vi "Spindle_load_RT_1 (SubVI).vi"(9 "?":T1, 10 "concatenated string 4":string, 11 "String":string) -> (0 "error out":errorcluster, 1 "content 4":string, 2 "content1 2":string, 3 "output cluster":T1, 4 "empty? 2":bool, 5 "concatenated string":string, 6 "load":string, 7 "concatenated string 2":string)   [LabVIEW 2017]
uses:
  MT_connect_data.ctl
  <vilib>/regexp/Match Regular Expression.xnode
  <vilib>/addons/internet/NI_InternetTK_Core_VIs.lvlib
panel:
  out "Position A 2":string
  out "content 7":string
  out "content 6":string
  out "after match":string
  out "Z_position":string
  out "Z_load":string
  out "Y_load":string
  out "X_position":string
  out "X_load":string
  out "Y_poistion":string
  out "K_position":string
  out "J_position":string
  out "I_position":string
  out "concatenated string 6":string
  out "content 3":string
  out "Position B":string
  out "B_load":string
  out "A_Load":string
  out "content 2":string
  out "concatenated string 5":string
  out "Position A":string
  out "Avail":string
  out "Tool_ID":string
  out "Program_name":string
  out "Controller_Mode":string
  out "Line_code":string
  out "program_status":string
  out "Block":string
  out "feeover":string
  out "Speedover":string
  out "path feedrate":string
  out "content":string
  out "error out 2":errorcluster
  out "spindle speed":string
  out "content 5":string
  out "empty? 3":bool
  out "after match 3":string
  out "content1 3":string
  out "concatenated string 3":string
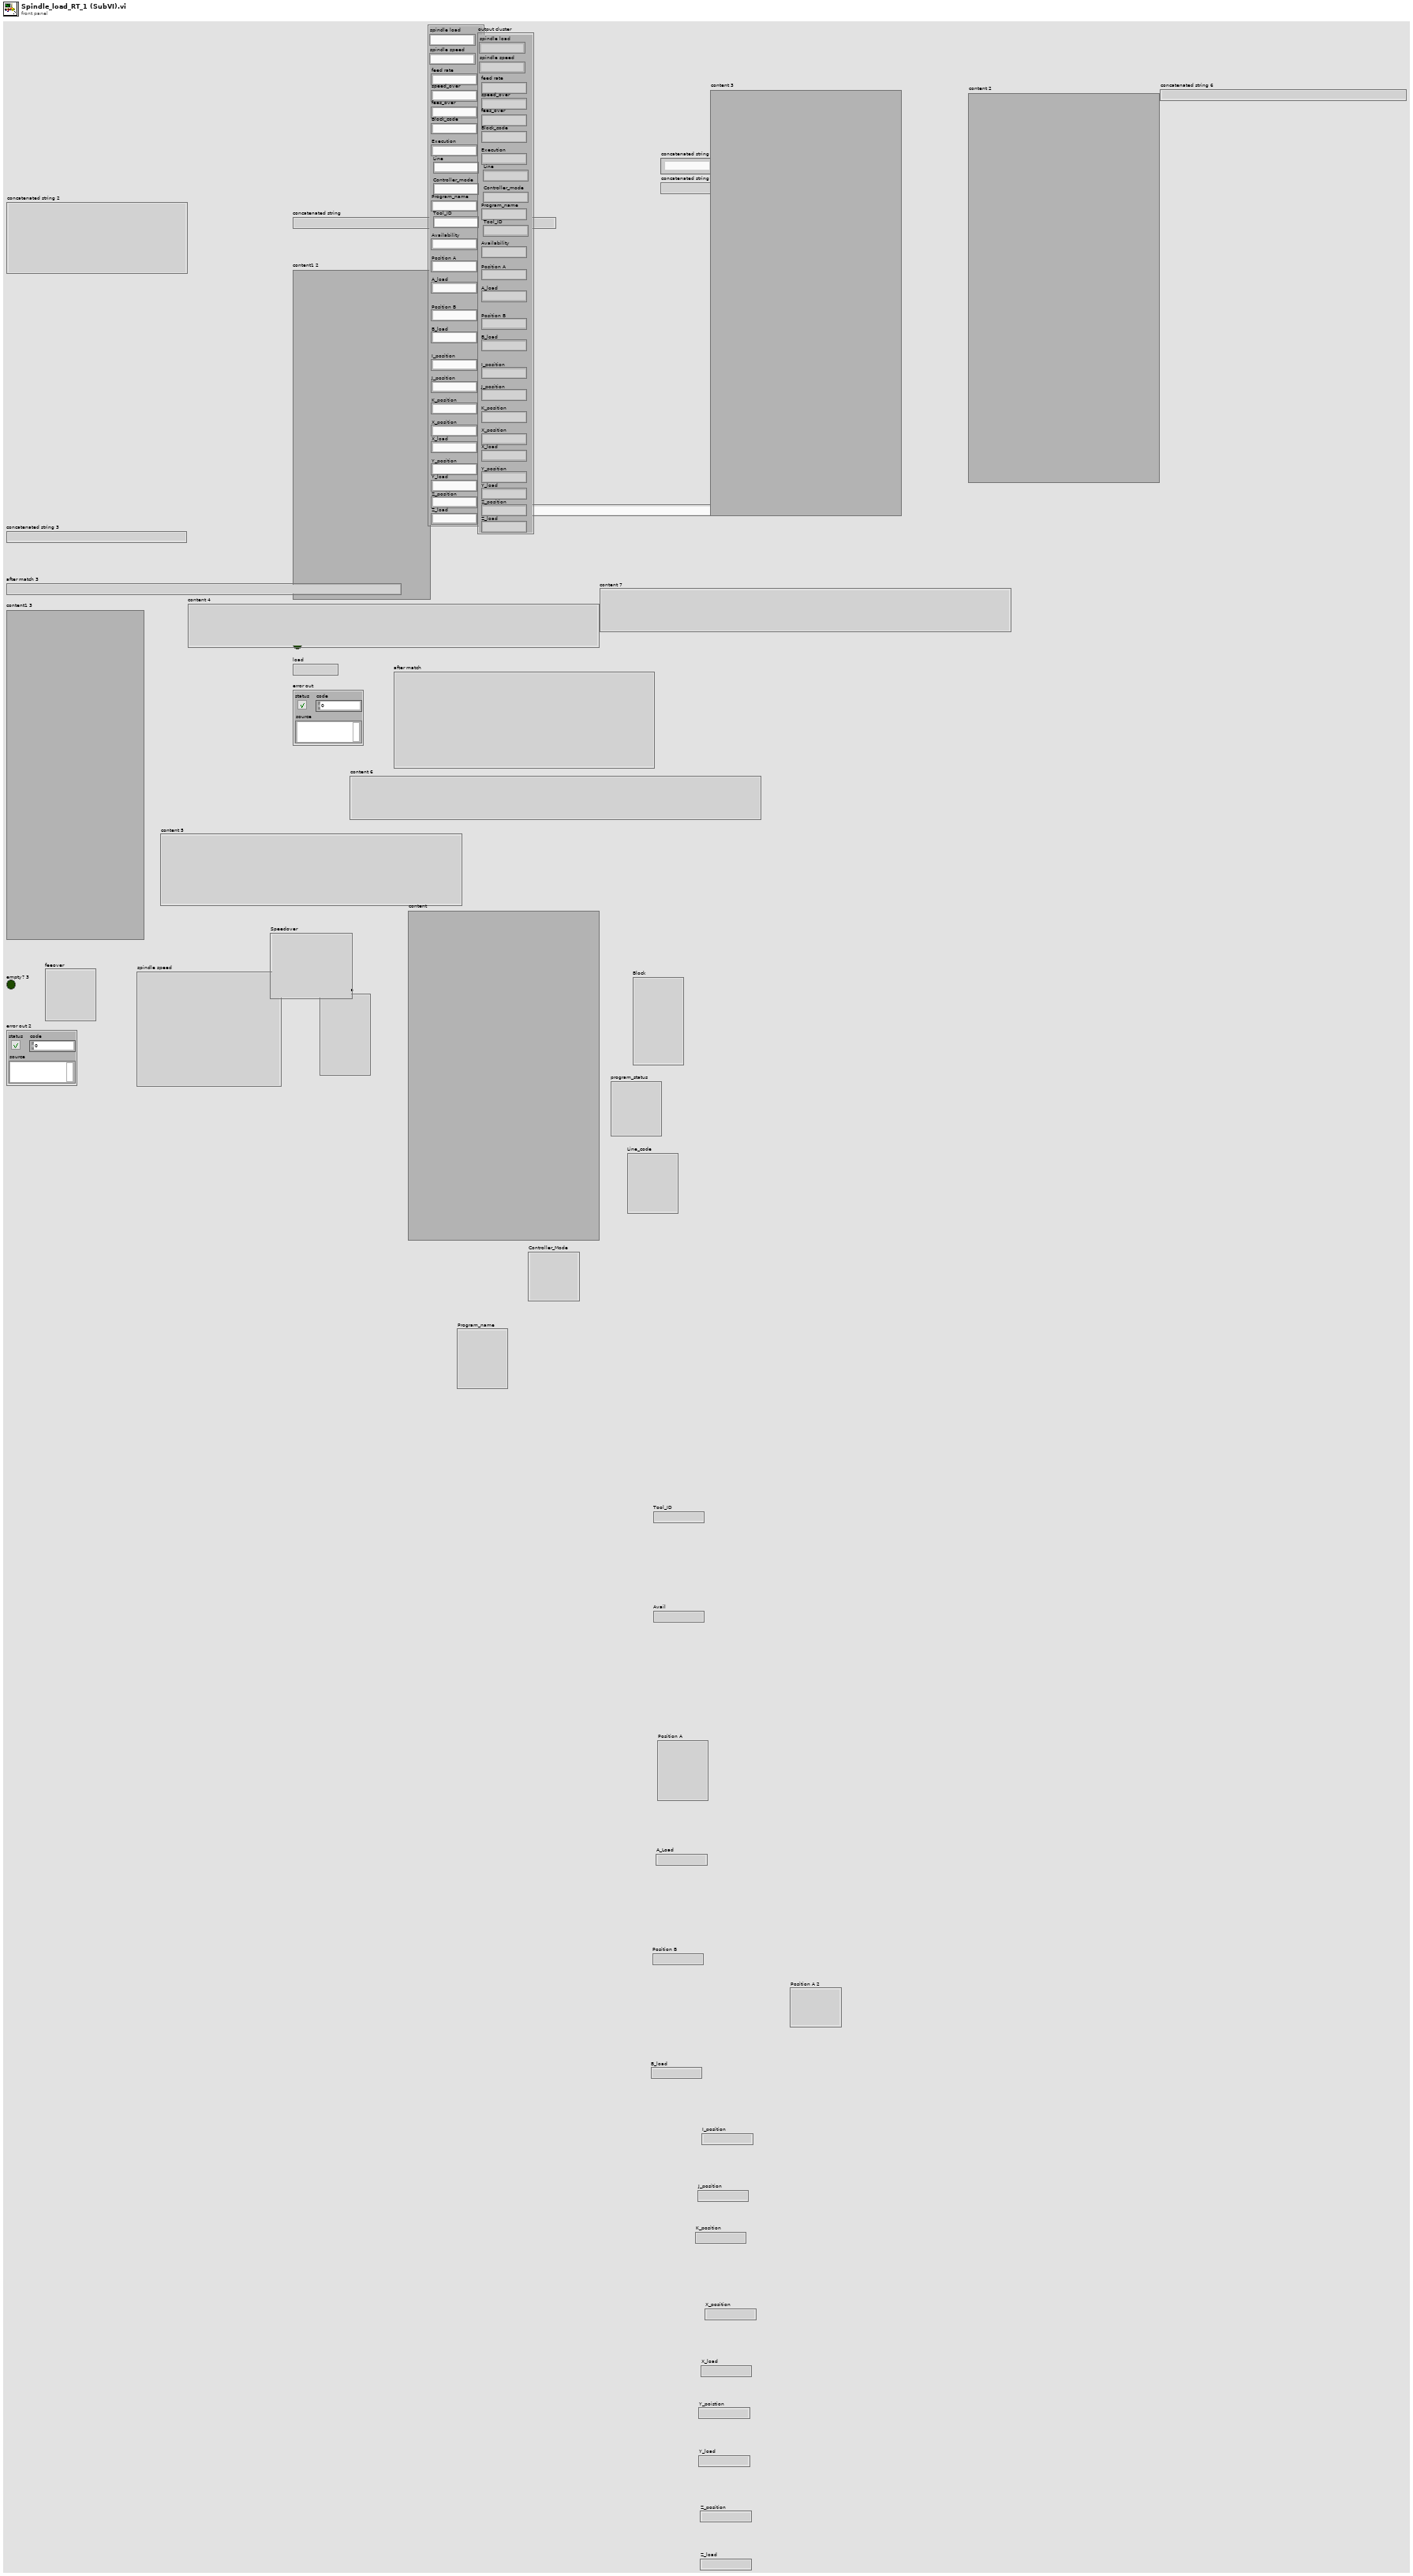
[diagram p1: front panel]
types:
  T1 = typedef "MT_connect_data.ctl" = cluster{"spindle load ":string, "spindle speed ":string, "feed rate":string, "speed_over":string, "fees_over":string, "Block_code":string, "Execution":string, "Line":string, "Controller_mode":string, "Program_name":string, "Tool_ID":string, "Availability":string, "Position A":string, "A_load":string, "Position B":string, "B_load":string, "I_position":string, "J_position":string, "K_position":string, "X_position":string, "X_load":string, "Y_position":string, "Y_load":string, "Z_position":string, "Z_load":string}
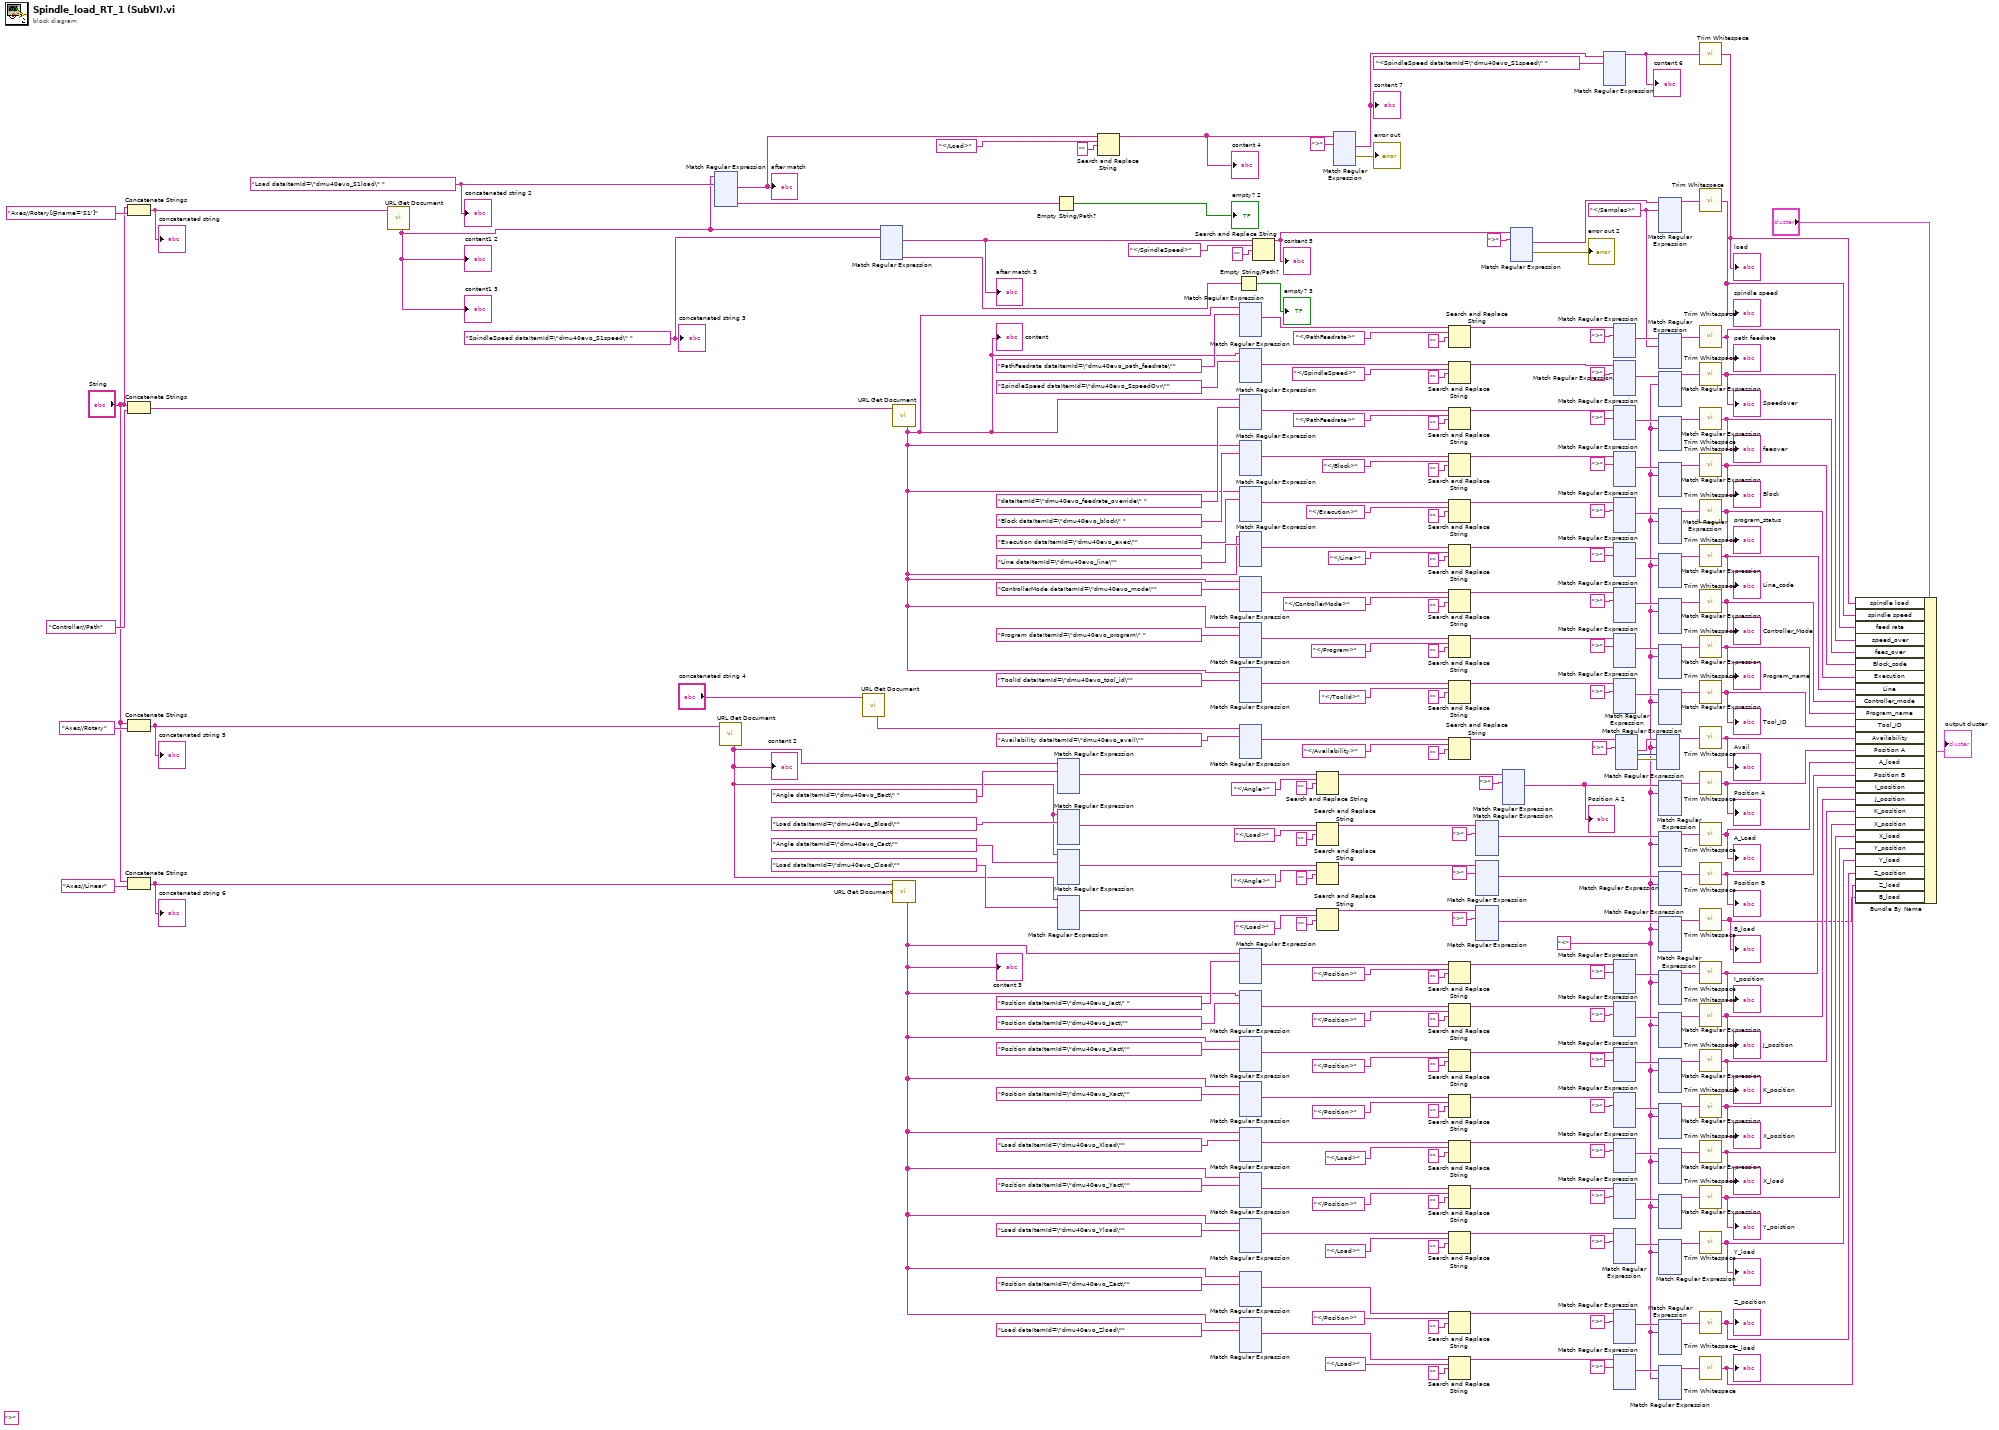
[diagram p0: block diagram]
diagram:
  w4 = "<" ("string")
  w55 = "</Samples>" ("string")
  (unwired) ">" ("string")
  w241 = "SpindleSpeed dataItemId=\"dmu40evo_S1speed\" " ("regular expression")
  w252 = "Load dataItemId=\"dmu40evo_S1load\" " ("regular expression")
  n1 = Concatenate Strings("String", "Axes//Rotary[@name='S1']" ("string")) -> (w247:string)
  "concatenated string" <- w247
  n2 = Concatenate Strings("String", "Controller//Path" ("string")) -> (w228:string)
  n3 = Concatenate Strings("String", "Axes//Rotary" ("string")) -> (w127:string)
  "concatenated string 5" <- w127
  n4 = Concatenate Strings("String", "Axes//Linear" ("string")) -> (w126:string)
  "concatenated string 6" <- w126
  n5 = call <vilib>:"URL Get Document.vi"("URL"=w247) -> ("content"=w233:string)  [unwired: 6 in, 4 out]
  "content1 2" <- w233
  "content1 3" <- w233
  n6 = xnode "Match Regular Expression"("input string"=w233, "regular expression"=w252) -> ("after match"=w244:string, "submatch 1"=w246:string)  [unwired: 4 in, 4 out]
  "after match" <- w244
  n7 = call <vilib>:"URL Get Document.vi"("URL"=w127) -> ("content"=w131:string)  [unwired: 6 in, 4 out]
  "content 2" <- w131
  n8 = call <vilib>:"URL Get Document.vi"("URL"="concatenated string 4") -> ("content"=w163:string)  [unwired: 6 in, 4 out]
  n9 = xnode "Match Regular Expression"("input string"=w233, "regular expression"=w241) -> ("after match"=w235:string, "submatch 1"=w237:string)  [unwired: 4 in, 4 out]
  "after match 3" <- w235
  n10 = call <vilib>:"URL Get Document.vi"("URL"=w228) -> ("content"=w162:string)  [unwired: 6 in, 4 out]
  "content" <- w162
  n11 = call <vilib>:"URL Get Document.vi"("URL"=w126) -> ("content"=w70:string)  [unwired: 6 in, 4 out]
  "content 3" <- w70
  n12 = Empty String/Path?(string/path=w246) -> (empty?=→"empty? 2":bool)
  n13 = xnode "Match Regular Expression"("input string"=w131, "regular expression"="Angle dataItemId=\"dmu40evo_Bact\" ") -> ("after match"=w155:string)  [unwired: 4 in, 5 out]
  n14 = xnode "Match Regular Expression"("input string"=w131, "regular expression"="Load dataItemId=\"dmu40evo_Bload\"") -> ("after match"=w145:string)  [unwired: 4 in, 5 out]
  n15 = xnode "Match Regular Expression"("input string"=w131, "regular expression"="Angle dataItemId=\"dmu40evo_Cact\"") -> ("after match"=w133:string)  [unwired: 4 in, 5 out]
  n16 = xnode "Match Regular Expression"("input string"=w131, "regular expression"="Load dataItemId=\"dmu40evo_Cload\"") -> ("after match"=w142:string)  [unwired: 4 in, 5 out]
  n17 = Search and Replace String(input string=w244, search string="</Load>" ("string"), replace string="" ("string")) -> (result string=w243:string)  [unwired: 5 in, 3 out]
  "content 4" <- w243
  n18 = Empty String/Path?(string/path=w237) -> (empty?=→"empty? 3":bool)
  n19 = xnode "Match Regular Expression"("input string"=w162, "regular expression"="PathFeedrate dataItemId=\"dmu40evo_path_feedrate\"") -> ("after match"=w226:string)  [unwired: 4 in, 5 out]
  n20 = xnode "Match Regular Expression"("input string"=w162, "regular expression"="SpindleSpeed dataItemId=\"dmu40evo_SspeedOvr\"") -> ("after match"=w214:string)  [unwired: 4 in, 5 out]
  n21 = xnode "Match Regular Expression"("input string"=w162, "regular expression"="dataItemId=\"dmu40evo_feedrate_override\" ") -> ("after match"=w213:string)  [unwired: 4 in, 5 out]
  n22 = xnode "Match Regular Expression"("input string"=w162, "regular expression"="Block dataItemId=\"dmu40evo_block\" ") -> ("after match"=w200:string)  [unwired: 4 in, 5 out]
  n23 = xnode "Match Regular Expression"("input string"=w162, "regular expression"="Execution dataItemId=\"dmu40evo_exec\"") -> ("after match"=w192:string)  [unwired: 4 in, 5 out]
  n24 = xnode "Match Regular Expression"("input string"=w162, "regular expression"="Line dataItemId=\"dmu40evo_line\"") -> ("after match"=w191:string)  [unwired: 4 in, 5 out]
  n25 = xnode "Match Regular Expression"("input string"=w162, "regular expression"="ControllerMode dataItemId=\"dmu40evo_mode\"") -> ("after match"=w187:string)  [unwired: 4 in, 5 out]
  n26 = xnode "Match Regular Expression"("input string"=w162, "regular expression"="Program dataItemId=\"dmu40evo_program\" ") -> ("after match"=w178:string)  [unwired: 4 in, 5 out]
  n27 = xnode "Match Regular Expression"("input string"=w162, "regular expression"="ToolId dataItemId=\"dmu40evo_tool_id\"") -> ("after match"=w175:string)  [unwired: 4 in, 5 out]
  n28 = xnode "Match Regular Expression"("input string"=w163, "regular expression"="Availability dataItemId=\"dmu40evo_avail\"") -> ("after match"=w166:string)  [unwired: 4 in, 5 out]
  n29 = xnode "Match Regular Expression"("input string"=w70, "regular expression"="Position dataItemId=\"dmu40evo_Iact\" ") -> ("after match"=w120:string)  [unwired: 4 in, 5 out]
  n30 = xnode "Match Regular Expression"("input string"=w70, "regular expression"="Position dataItemId=\"dmu40evo_Jact\"") -> ("after match"=w117:string)  [unwired: 4 in, 5 out]
  n31 = xnode "Match Regular Expression"("input string"=w70, "regular expression"="Position dataItemId=\"dmu40evo_Kact\"") -> ("after match"=w108:string)  [unwired: 4 in, 5 out]
  n32 = xnode "Match Regular Expression"("input string"=w70, "regular expression"="Position dataItemId=\"dmu40evo_Xact\"") -> ("after match"=w93:string)  [unwired: 4 in, 5 out]
  n33 = xnode "Match Regular Expression"("input string"=w70, "regular expression"="Load dataItemId=\"dmu40evo_Xload\"") -> ("after match"=w96:string)  [unwired: 4 in, 5 out]
  n34 = xnode "Match Regular Expression"("input string"=w70, "regular expression"="Position dataItemId=\"dmu40evo_Yact\"") -> ("after match"=w105:string)  [unwired: 4 in, 5 out]
  n35 = xnode "Match Regular Expression"("input string"=w70, "regular expression"="Load dataItemId=\"dmu40evo_Yload\"") -> ("after match"=w84:string)  [unwired: 4 in, 5 out]
  n36 = xnode "Match Regular Expression"("input string"=w70, "regular expression"="Position dataItemId=\"dmu40evo_Zact\"") -> ("after match"=w72:string)  [unwired: 4 in, 5 out]
  n37 = xnode "Match Regular Expression"("input string"=w70, "regular expression"="Load dataItemId=\"dmu40evo_Zload\"") -> ("after match"=w81:string)  [unwired: 4 in, 5 out]
  n38 = Search and Replace String(input string=w235, search string="</SpindleSpeed>" ("string"), replace string="" ("string")) -> (result string=w234:string)  [unwired: 5 in, 3 out]
  "content 5" <- w234
  n39 = Search and Replace String(input string=w155, search string="</Angle>" ("string"), replace string="" ("string")) -> (result string=w156:string)  [unwired: 5 in, 3 out]
  n40 = Search and Replace String(input string=w145, search string="</Load>" ("string"), replace string="" ("string")) -> (result string=w144:string)  [unwired: 5 in, 3 out]
  n41 = Search and Replace String(input string=w133, search string="</Angle>" ("string"), replace string="" ("string")) -> (result string=w132:string)  [unwired: 5 in, 3 out]
  n42 = Search and Replace String(input string=w142, search string="</Load>" ("string"), replace string="" ("string")) -> (result string=w143:string)  [unwired: 5 in, 3 out]
  n43 = xnode "Match Regular Expression"("input string"=w243, "regular expression"=">" ("string")) -> ("after match"=w59:string, "error out"=→"error out":errorcluster)  [unwired: 4 in, 4 out]
  "content 7" <- w59
  n44 = Search and Replace String(input string=w226, search string="</PathFeedrate>" ("string"), replace string="" ("string")) -> (result string=w221:string)  [unwired: 5 in, 3 out]
  n45 = Search and Replace String(input string=w214, search string="</SpindleSpeed>" ("string"), replace string="" ("string")) -> (result string=w219:string)  [unwired: 5 in, 3 out]
  n46 = Search and Replace String(input string=w213, search string="</PathFeedrate>" ("string"), replace string="" ("string")) -> (result string=w208:string)  [unwired: 5 in, 3 out]
  n47 = Search and Replace String(input string=w200, search string="</Block>" ("string"), replace string="" ("string")) -> (result string=w205:string)  [unwired: 5 in, 3 out]
  n48 = Search and Replace String(input string=w192, search string="</Execution>" ("string"), replace string="" ("string")) -> (result string=w190:string)  [unwired: 5 in, 3 out]
  n49 = Search and Replace String(input string=w191, search string="</Line>" ("string"), replace string="" ("string")) -> (result string=w189:string)  [unwired: 5 in, 3 out]
  n50 = Search and Replace String(input string=w187, search string="</ControllerMode>" ("string"), replace string="" ("string")) -> (result string=w188:string)  [unwired: 5 in, 3 out]
  n51 = Search and Replace String(input string=w178, search string="</Program>" ("string"), replace string="" ("string")) -> (result string=w177:string)  [unwired: 5 in, 3 out]
  n52 = Search and Replace String(input string=w175, search string="</ToolId>" ("string"), replace string="" ("string")) -> (result string=w176:string)  [unwired: 5 in, 3 out]
  n53 = Search and Replace String(input string=w166, search string="</Availability>" ("string"), replace string="" ("string")) -> (result string=w165:string)  [unwired: 5 in, 3 out]
  n54 = Search and Replace String(input string=w120, search string="</Position>" ("string"), replace string="" ("string")) -> (result string=w119:string)  [unwired: 5 in, 3 out]
  n55 = Search and Replace String(input string=w117, search string="</Position>" ("string"), replace string="" ("string")) -> (result string=w118:string)  [unwired: 5 in, 3 out]
  n56 = Search and Replace String(input string=w108, search string="</Position>" ("string"), replace string="" ("string")) -> (result string=w107:string)  [unwired: 5 in, 3 out]
  n57 = Search and Replace String(input string=w93, search string="</Position>" ("string"), replace string="" ("string")) -> (result string=w94:string)  [unwired: 5 in, 3 out]
  n58 = Search and Replace String(input string=w96, search string="</Load>" ("string"), replace string="" ("string")) -> (result string=w95:string)  [unwired: 5 in, 3 out]
  n59 = Search and Replace String(input string=w105, search string="</Position>" ("string"), replace string="" ("string")) -> (result string=w106:string)  [unwired: 5 in, 3 out]
  n60 = Search and Replace String(input string=w84, search string="</Load>" ("string"), replace string="" ("string")) -> (result string=w83:string)  [unwired: 5 in, 3 out]
  n61 = Search and Replace String(input string=w72, search string="</Position>" ("string"), replace string="" ("string")) -> (result string=w71:string)  [unwired: 5 in, 3 out]
  n62 = Search and Replace String(input string=w81, search string="</Load>" ("string"), replace string="" ("string")) -> (result string=w82:string)  [unwired: 5 in, 3 out]
  n63 = xnode "Match Regular Expression"("input string"=w144, "regular expression"=">" ("string")) -> ("after match"=w35:string)  [unwired: 4 in, 5 out]
  n64 = xnode "Match Regular Expression"("input string"=w132, "regular expression"=">" ("string")) -> ("after match"=w34:string)  [unwired: 4 in, 5 out]
  n65 = xnode "Match Regular Expression"("input string"=w143, "regular expression"=">" ("string")) -> ("after match"=w33:string)  [unwired: 4 in, 5 out]
  n66 = xnode "Match Regular Expression"("input string"=w156, "regular expression"=">" ("string")) -> ("after match"=w23:string)  [unwired: 4 in, 5 out]
  "Position A 2" <- w23
  n67 = xnode "Match Regular Expression"("input string"=w234, "regular expression"=">" ("string")) -> ("after match"=w58:string, "error out"=→"error out 2":errorcluster)  [unwired: 4 in, 4 out]
  n68 = xnode "Match Regular Expression"("input string"=w59, "regular expression"="<SpindleSpeed dataItemId=\"dmu40evo_S1speed\" ") -> ("before match"=w60:string)  [unwired: 4 in, 5 out]
  "content 6" <- w60
  n69 = xnode "Match Regular Expression"("input string"=w221, "regular expression"=">" ("string")) -> ("after match"=w56:string)  [unwired: 4 in, 5 out]
  n70 = xnode "Match Regular Expression"("input string"=w219, "regular expression"=">" ("string")) -> ("after match"=w49:string)  [unwired: 4 in, 5 out]
  n71 = xnode "Match Regular Expression"("input string"=w208, "regular expression"=">" ("string")) -> ("after match"=w5:string)  [unwired: 4 in, 5 out]
  n72 = xnode "Match Regular Expression"("input string"=w205, "regular expression"=">" ("string")) -> ("after match"=w8:string)  [unwired: 4 in, 5 out]
  n73 = xnode "Match Regular Expression"("input string"=w190, "regular expression"=">" ("string")) -> ("after match"=w51:string)  [unwired: 4 in, 5 out]
  n74 = xnode "Match Regular Expression"("input string"=w189, "regular expression"=">" ("string")) -> ("after match"=w47:string)  [unwired: 4 in, 5 out]
  n75 = xnode "Match Regular Expression"("input string"=w188, "regular expression"=">" ("string")) -> ("after match"=w45:string)  [unwired: 4 in, 5 out]
  n76 = xnode "Match Regular Expression"("input string"=w177, "regular expression"=">" ("string")) -> ("after match"=w39:string)  [unwired: 4 in, 5 out]
  n77 = xnode "Match Regular Expression"("input string"=w176, "regular expression"=">" ("string")) -> ("after match"=w38:string)  [unwired: 4 in, 5 out]
  n78 = xnode "Match Regular Expression"("input string"=w119, "regular expression"=">" ("string")) -> ("after match"=w32:string)  [unwired: 4 in, 5 out]
  n79 = xnode "Match Regular Expression"("input string"=w118, "regular expression"=">" ("string")) -> ("after match"=w31:string)  [unwired: 4 in, 5 out]
  n80 = xnode "Match Regular Expression"("input string"=w107, "regular expression"=">" ("string")) -> ("after match"=w30:string)  [unwired: 4 in, 5 out]
  n81 = xnode "Match Regular Expression"("input string"=w94, "regular expression"=">" ("string")) -> ("after match"=w29:string)  [unwired: 4 in, 5 out]
  n82 = xnode "Match Regular Expression"("input string"=w95, "regular expression"=">" ("string")) -> ("after match"=w28:string)  [unwired: 4 in, 5 out]
  n83 = xnode "Match Regular Expression"("input string"=w106, "regular expression"=">" ("string")) -> ("after match"=w27:string)  [unwired: 4 in, 5 out]
  n84 = xnode "Match Regular Expression"("input string"=w83, "regular expression"=">" ("string")) -> ("after match"=w26:string)  [unwired: 4 in, 5 out]
  n85 = xnode "Match Regular Expression"("input string"=w71, "regular expression"=">" ("string")) -> ("after match"=w25:string)  [unwired: 4 in, 5 out]
  n86 = xnode "Match Regular Expression"("input string"=w82, "regular expression"=">" ("string")) -> ("after match"=w24:string)  [unwired: 4 in, 5 out]
  n87 = xnode "Match Regular Expression"("input string"=w165, "regular expression"=">" ("string")) -> ("after match"=w37:string, "offset past match"=w41:i32, "error out"=w40:errorcluster)  [unwired: 4 in, 3 out]
  n88 = xnode "Match Regular Expression"("input string"=w37, "regular expression"=w4, "offset (0)"=w41, "error in"=w40) -> ("before match"=w22:string)  [unwired: 2 in, 5 out]
  n89 = xnode "Match Regular Expression"("input string"=w58, "regular expression"=w55) -> ("before match"=w57:string)  [unwired: 4 in, 5 out]
  n90 = xnode "Match Regular Expression"("input string"=w56, "regular expression"=w55) -> ("before match"=w54:string)  [unwired: 4 in, 5 out]
  n91 = xnode "Match Regular Expression"("input string"=w49, "regular expression"=w4) -> ("before match"=w53:string)  [unwired: 4 in, 5 out]
  n92 = xnode "Match Regular Expression"("input string"=w5, "regular expression"=w4) -> ("before match"=w6:string)  [unwired: 4 in, 5 out]
  n93 = xnode "Match Regular Expression"("input string"=w8, "regular expression"=w4) -> ("before match"=w7:string)  [unwired: 4 in, 5 out]
  n94 = xnode "Match Regular Expression"("input string"=w51, "regular expression"=w4) -> ("before match"=w50:string)  [unwired: 4 in, 5 out]
  n95 = xnode "Match Regular Expression"("input string"=w47, "regular expression"=w4) -> ("before match"=w46:string)  [unwired: 4 in, 5 out]
  n96 = xnode "Match Regular Expression"("input string"=w45, "regular expression"=w4) -> ("before match"=w44:string)  [unwired: 4 in, 5 out]
  n97 = xnode "Match Regular Expression"("input string"=w39, "regular expression"=w4) -> ("before match"=w43:string)  [unwired: 4 in, 5 out]
  n98 = xnode "Match Regular Expression"("input string"=w38, "regular expression"=w4) -> ("before match"=w42:string)  [unwired: 4 in, 5 out]
  n99 = xnode "Match Regular Expression"("input string"=w23, "regular expression"=w4) -> ("before match"=w21:string)  [unwired: 4 in, 5 out]
  n100 = xnode "Match Regular Expression"("input string"=w35, "regular expression"=w4) -> ("before match"=w20:string)  [unwired: 4 in, 5 out]
  n101 = xnode "Match Regular Expression"("input string"=w34, "regular expression"=w4) -> ("before match"=w19:string)  [unwired: 4 in, 5 out]
  n102 = xnode "Match Regular Expression"("input string"=w33, "regular expression"=w4) -> ("before match"=w18:string)  [unwired: 4 in, 5 out]
  n103 = xnode "Match Regular Expression"("input string"=w32, "regular expression"=w4) -> ("before match"=w17:string)  [unwired: 4 in, 5 out]
  n104 = xnode "Match Regular Expression"("input string"=w31, "regular expression"=w4) -> ("before match"=w16:string)  [unwired: 4 in, 5 out]
  n105 = xnode "Match Regular Expression"("input string"=w30, "regular expression"=w4) -> ("before match"=w15:string)  [unwired: 4 in, 5 out]
  n106 = xnode "Match Regular Expression"("input string"=w29, "regular expression"=w4) -> ("before match"=w14:string)  [unwired: 4 in, 5 out]
  n107 = xnode "Match Regular Expression"("input string"=w28, "regular expression"=w4) -> ("before match"=w13:string)  [unwired: 4 in, 5 out]
  n108 = xnode "Match Regular Expression"("input string"=w27, "regular expression"=w4) -> ("before match"=w12:string)  [unwired: 4 in, 5 out]
  n109 = xnode "Match Regular Expression"("input string"=w26, "regular expression"=w4) -> ("before match"=w11:string)  [unwired: 4 in, 5 out]
  n110 = xnode "Match Regular Expression"("input string"=w25, "regular expression"=w4) -> ("before match"=w10:string)  [unwired: 4 in, 5 out]
  n111 = xnode "Match Regular Expression"("input string"=w24, "regular expression"=w4) -> ("before match"=w9:string)  [unwired: 4 in, 5 out]
  n112 = call <vilib>:"Trim Whitespace.vi"("string"=w60) -> ("trimmed string"=w231:string)  [unwired: 1 in]
  "load" <- w231
  n113 = call <vilib>:"Trim Whitespace.vi"("string"=w57) -> ("trimmed string"=w230:string)  [unwired: 1 in]
  "spindle speed" <- w230
  n114 = call <vilib>:"Trim Whitespace.vi"("string"=w54) -> ("trimmed string"=w220:string)  [unwired: 1 in]
  "path feedrate" <- w220
  n115 = call <vilib>:"Trim Whitespace.vi"("string"=w53) -> ("trimmed string"=w207:string)  [unwired: 1 in]
  "Speedover" <- w207
  n116 = call <vilib>:"Trim Whitespace.vi"("string"=w6) -> ("trimmed string"=w206:string)  [unwired: 1 in]
  "feeover" <- w206
  n117 = call <vilib>:"Trim Whitespace.vi"("string"=w7) -> ("trimmed string"=w3:string)  [unwired: 1 in]
  "Block" <- w3
  n118 = call <vilib>:"Trim Whitespace.vi"("string"=w50) -> ("trimmed string"=w161:string)  [unwired: 1 in]
  "program_status" <- w161
  n119 = call <vilib>:"Trim Whitespace.vi"("string"=w46) -> ("trimmed string"=w48:string)  [unwired: 1 in]
  "Line_code" <- w48
  n120 = call <vilib>:"Trim Whitespace.vi"("string"=w44) -> ("trimmed string"=w160:string)  [unwired: 1 in]
  "Controller_Mode" <- w160
  n121 = call <vilib>:"Trim Whitespace.vi"("string"=w43) -> ("trimmed string"=w159:string)  [unwired: 1 in]
  "Program_name" <- w159
  n122 = call <vilib>:"Trim Whitespace.vi"("string"=w42) -> ("trimmed string"=w158:string)  [unwired: 1 in]
  "Tool_ID" <- w158
  n123 = call <vilib>:"Trim Whitespace.vi"("string"=w22) -> ("trimmed string"=w157:string)  [unwired: 1 in]
  "Avail" <- w157
  n124 = call <vilib>:"Trim Whitespace.vi"("string"=w21) -> ("trimmed string"=w130:string)  [unwired: 1 in]
  "Position A" <- w130
  n125 = call <vilib>:"Trim Whitespace.vi"("string"=w20) -> ("trimmed string"=w36:string)  [unwired: 1 in]
  "A_Load" <- w36
  n126 = call <vilib>:"Trim Whitespace.vi"("string"=w19) -> ("trimmed string"=w129:string)  [unwired: 1 in]
  "Position B" <- w129
  n127 = call <vilib>:"Trim Whitespace.vi"("string"=w18) -> ("trimmed string"=w2:string)  [unwired: 1 in]
  "B_load" <- w2
  n128 = call <vilib>:"Trim Whitespace.vi"("string"=w17) -> ("trimmed string"=w1:string)  [unwired: 1 in]
  "I_position" <- w1
  n129 = call <vilib>:"Trim Whitespace.vi"("string"=w16) -> ("trimmed string"=w69:string)  [unwired: 1 in]
  "J_position" <- w69
  n130 = call <vilib>:"Trim Whitespace.vi"("string"=w15) -> ("trimmed string"=w68:string)  [unwired: 1 in]
  "K_position" <- w68
  n131 = call <vilib>:"Trim Whitespace.vi"("string"=w14) -> ("trimmed string"=w67:string)  [unwired: 1 in]
  "X_position" <- w67
  n132 = call <vilib>:"Trim Whitespace.vi"("string"=w13) -> ("trimmed string"=w66:string)  [unwired: 1 in]
  "X_load" <- w66
  n133 = call <vilib>:"Trim Whitespace.vi"("string"=w12) -> ("trimmed string"=w65:string)  [unwired: 1 in]
  "Y_poistion" <- w65
  n134 = call <vilib>:"Trim Whitespace.vi"("string"=w11) -> ("trimmed string"=w64:string)  [unwired: 1 in]
  "Y_load" <- w64
  n135 = call <vilib>:"Trim Whitespace.vi"("string"=w10) -> ("trimmed string"=w63:string)  [unwired: 1 in]
  "Z_position" <- w63
  n136 = call <vilib>:"Trim Whitespace.vi"("string"=w9) -> ("trimmed string"=w62:string)  [unwired: 1 in]
  "Z_load" <- w62
  n137 = Bundle By Name(cluster="?", "spindle load"=w231, "spindle speed"=w230, "feed rate"=w220, "speed_over"=w207, "fees_over"=w206, "Block_code"=w3, "Execution"=w161, "Line"=w48, "Controller_mode"=w160, "Program_name"=w159, "Tool_ID"=w158, "Availability"=w157, "Position A"=w130, "A_load"=w36, "Position B"=w129, "I_position"=w1, "J_position"=w69, "K_position"=w68, "X_position"=w67, "X_load"=w66, "Y_position"=w65, "Y_load"=w64, "Z_position"=w63, "Z_load"=w62, "B_load"=w2) -> (→"output cluster":T1)
  "concatenated string 2" <- w252
  "concatenated string 3" <- w241
